vi "UT_EField_DAQ_AnalogIO.set device ID.vi"(0 "i ref in":refnum<vi>, 3 "Timeout":i32=10000, 5 "error in":errorcluster caption="Fehler (Eingang, kein Fehler)") -> (14 "i ref out":refnum<vi>, 17 "timed out":bool, 19 "error out":errorcluster caption="Fehler (Ausgang)")   [LabVIEW 2014, in "UT_EField_DAQ_AnalogIO.lvlib"]
doc: "Contact: Falk Ziegler, eMail: info@lab-coding.de"
uses:
  UT_EField_DAQ_AnalogIO.lvlib
  CS_Core/BaseProcess/BaseProcess.lvlib
  CS_Core/CSApplicationBaseClasses/DeviceBase/DeviceBase.lvlib
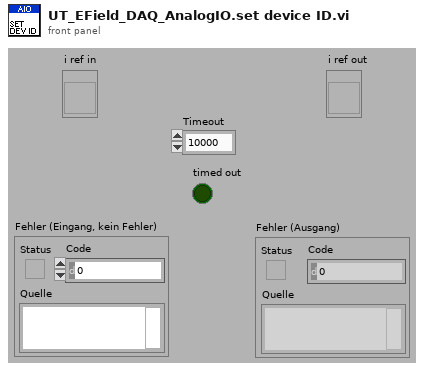
[diagram p1: front panel]
types:
  T1 = typedef "BaseProcess.lvlib/BaseProcess.i attribute.ctl" = cluster{"EventStatus":string, "EventError":i32, "PresetEvtWatchD":i32, "PresetPdcWatchD":i32, "EventTimeout":i32, "PeriodicInterval":i32, "Interface":string[], "Address":string[], "Special":string[], "PeriodicError":i32, "PeriodicStatus":string, "SuperProc":string, "Descriptors":T2[], "CaseRef":refnum<vi>, "PdcRef":refnum<vi>, "Thread Ref":refnum<vi>, "eventErrorID":i32, "eventStatusID":i32, "periodicErrorID":i32, "periodicStatusID":i32, "pdcCtrID":i32}
  T2 = typedef "BaseProcess.lvlib/BaseProcess.descriptor definition.ctl" = cluster{"selector":string, "descriptor":T3}
  T3 = typedef "BaseProcess.lvlib/BaseProcess.descriptor string definition.ctl" = string
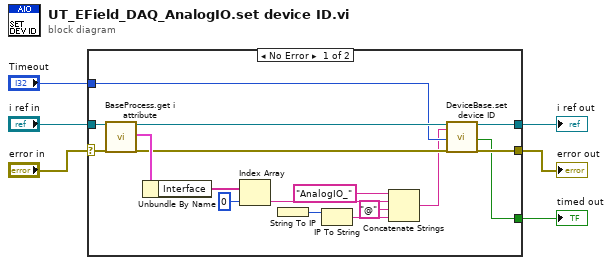
[diagram p0: block diagram]
diagram:
  n1 = case shown="No Error" "error in" {
    selector: "error in" -> [w22 w25]
    tunnel: "i ref in" -> [w23 w24]
    tunnel: [w8 w25] -> w4
    tunnel: [w9 w24] -> w3
    tunnel: "Timeout" -> [w11 _]
    tunnel: [w7 _] -> w1
    frame No Error {
      n2 = call "BaseProcess.get i attribute.vi"("i ref in"=w23, "error in (no error)"=w22) -> ("i ref out"=w18:refnum<vi>, "i attribute"=w21:T1, "error out"=w17:errorcluster)  [unwired: 15 in]
      n3 = Unbundle By Name(w21) -> ("Interface"=w20:string[])
      n4 = Index Array(array=w20, index=0 ("Index")) -> (element=w14:string)
      n5 = String To IP() -> (0:w13:u32)  [unwired: 1 in]
      n6 = IP To String(2:w13) -> (0:w12:string)  [unwired: 1 in]
      n7 = Concatenate Strings("AnalogIO_", w14, "@" ("String"), w12) -> (w10:string)
      n8 = call "DeviceBase.set device ID.vi"("i ref in"=w18, "deviceID"=w10, "ms timeout (10000)"=w11, "error in (no error)"=w17) -> ("i ref out"=w9:refnum<vi>, "timed out"=w7:bool, "error out"=w8:errorcluster)  [unwired: 13 in]
    }
    frame Error {
    }
  }
  "error out" <- w4
  "timed out" <- w1
  "i ref out" <- w3
